vi "Update In World.vi"(11 "Movable in":refnum<class "Element.lvclass">) -> (3 "Movable out":refnum<class "Element.lvclass">)   [LabVIEW 2015, in "Element.lvclass"]
uses:
  Element.lvclass
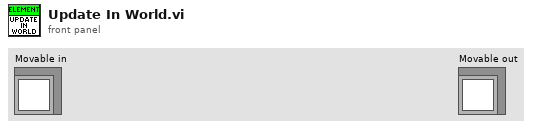
[diagram p1: front panel]
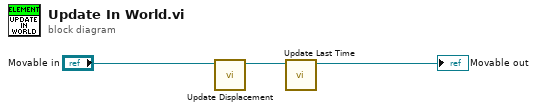
[diagram p0: block diagram]
diagram:
  n1 = call "Update Displacement.vi"("Movable in"="Movable in") -> ("Movable out"=w3:refnum<class "Element.lvclass">)  [unwired: 10 in]
  n2 = call "Update Last Time.vi"("Movable in"=w3) -> ("Movable out"=→"Movable out":refnum<class "Element.lvclass">)  [unwired: 10 in]
